vi "FSTOP_Powerstage_v1.vi"() -> (0 "error out":errorcluster, 3 "output string":string)   [LabVIEW 2022 SP3]
uses:
  <vilib>/Instr/_visa.llb/VISA Flush IO Buffer Mask.ctl
  <vilib>/DAQmx/write.llb/DAQmx Write (Digital 1D Bool NChan 1Samp 1Line).vi
  <vilib>/DAQmx/miscellaneous.llb/DAQmx Fill In Error Info.vi
panel:
  in  "error in (no error)":errorcluster
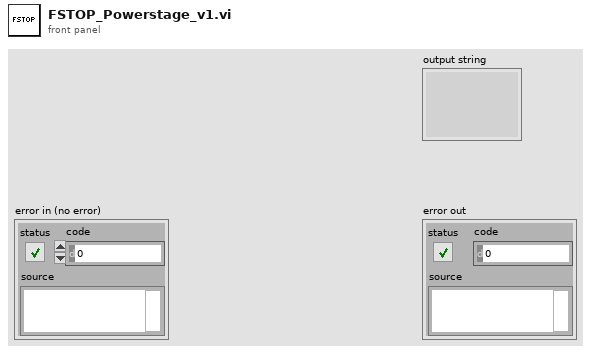
[diagram p1: front panel]
types:
  T1 = typedef "VISA Flush IO Buffer Mask.ctl" = u16
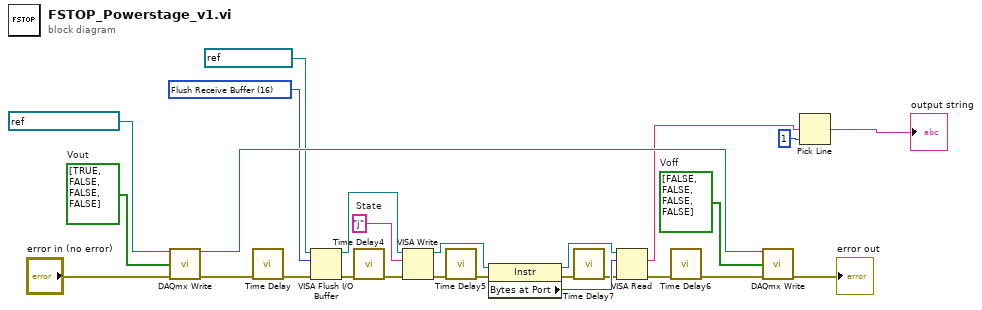
[diagram p0: block diagram]
diagram:
  w13 = "j"  # State
  w12 = bool[] [FALSE, FALSE, FALSE, FALSE]  # Voff
  w14 = bool[] [TRUE, FALSE, FALSE, FALSE]  # Vout
  w16 = T1 16 items=["Flush Receive Buffer"=16, "Write Transmit Buffer to Device"=32, "Flush Receive Buffer (No I/O)"=64, "Flush Transmit Buffer"=128] ("Mask")
  n1 = call-poly <vilib>:"DAQmx Write.vi"("task/channels in"=refnum<k21> "FTS2_DigitalOut", "data"=w14, "error in"="error in (no error)") -> ("task out"=w22:refnum<k21>, "error out"=w11:errorcluster)  [unwired: 10 in, 1 out]
  n2 = call "Time Delay"("error in (no error)"=w11) -> ("error out"=w10:errorcluster)  [unwired: 10 in]
  n3 = VISA Flush I/O Buffer(VISA resource name=refnum<visa-resource-name> "ControlBoard", mask (16)=w16, error in (no error)=w10) -> (VISA resource name out=w18:refnum<visa-resource-name>, error out=w15:errorcluster)
  n4 = call "Time Delay4"("error in (no error)"=w15) -> ("error out"=w26:errorcluster)  [unwired: 10 in]
  n5 = VISA Write(VISA resource name=w18, write buffer=w13, error in (no error)=w26) -> (VISA resource name out=w21:refnum<visa-resource-name>, error out=w7:errorcluster)  [unwired: 1 out]
  n6 = call "Time Delay5"("error in (no error)"=w7) -> ("error out"=w6:errorcluster)  [unwired: 10 in]
  n7 = property class="Instr"(reference=w21, error in=w6) -> (reference out=w20:refnum<visa-resource-name>, error out=w5:errorcluster, "Bytes at Port"=w19:u32)
  n8 = call "Time Delay7"("error in (no error)"=w5) -> ("error out"=w4:errorcluster)  [unwired: 10 in]
  n9 = VISA Read(VISA resource name=w20, byte count=w19, error in (no error)=w4) -> (read buffer=w1:string, error out=w24:errorcluster)  [unwired: 2 out]
  n10 = call "Time Delay6"("error in (no error)"=w24) -> ("error out"=w23:errorcluster)  [unwired: 10 in]
  n11 = call-poly <vilib>:"DAQmx Write.vi"("task/channels in"=w22, "data"=w12, "error in"=w23) -> ("error out"=→"error out":errorcluster)  [unwired: 10 in, 2 out]
  n12 = Pick Line(multi-line string=w1, line index=1) -> (output string=→"output string":string)  [unwired: 1 in]
